vi "Get all NodePath.vi"(8 "error in (no error)":errorcluster caption="错误输入（无错误）", 11 "PanelLinkNode 输入":refnum<class "PanelLinkNode.lvclass"> caption="DNL_LabVIEW Object in") -> (0 "error out":errorcluster caption="错误输出", 2 "All NodePath":string[](array[string]), 3 "PanelLinkNode 输出":refnum<class "PanelLinkNode.lvclass"> caption="DNL_LabVIEW Object out")   [LabVIEW 2016, in "PanelLinkNode.lvclass"]
uses:
  PanelLinkNode.lvclass
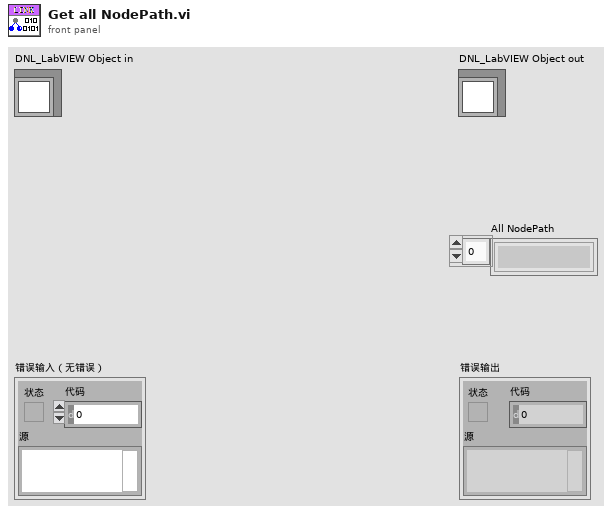
[diagram p1: front panel]
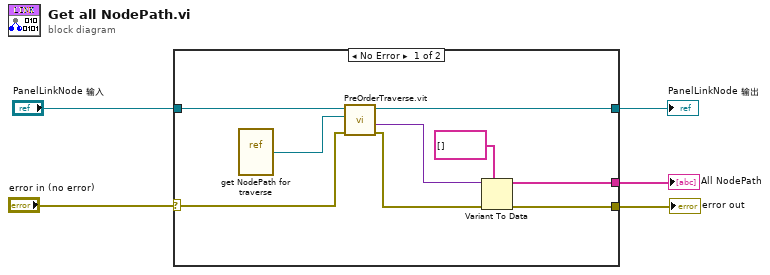
[diagram p0: block diagram]
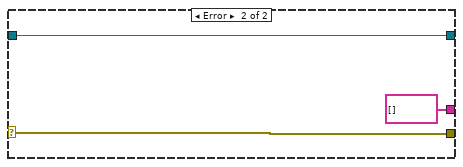
[diagram p2: hidden frame]
diagram:
  n1 = case shown="No Error" "error in (no error)" {
    selector: "error in (no error)" -> [w6 w17]
    tunnel: [w8 w17] -> w4
    tunnel: [w13 w16] -> w2
    tunnel: "PanelLinkNode 输入" -> [w14 w16]
    tunnel: [w7 string[] []] -> w1
    frame No Error {
      n2 = vi-ref "get NodePath for traverse.vi"() -> (w12:refnum<vi>)
      n3 = call-dynamic "PreOrderTraverse.vit"("error in"=w6, "vi reference"=w12, "PanelLinkNode 输入"=w14) -> ("error out"=w9:errorcluster, "Data out"=w11:variant, "PanelLinkNode 输出"=w13:refnum<class "PanelLinkNode.lvclass">)  [unwired: 5 in, 1 out]
      n4 = Variant To Data(error in=w9, type=string[] [], Variant=w11) -> (data=w7:string[], error out=w8:errorcluster)
    }
    frame Error {
    }
  }
  "error out" <- w4
  "PanelLinkNode 输出" <- w2
  "All NodePath" <- w1
